vi "PH_Sequencer.Switch PU FR on automatically.vi"(0 "i ref in":refnum<vi>, 5 "error in":errorcluster) -> (14 "i ref out":refnum<vi>, 19 "error out":errorcluster)   [LabVIEW 2014, in "PH_Sequencer.lvlib"]
doc: "This is the action done when PU SM States are changing."
uses:
  PH_Sequencer.lvlib
  PH_PP_Common/PH_PP_Common.PUs.ctl
  PH_BeamlineInformation/PH_BeamlineInformation.lvlib
  PH_PP_Common/PH_PP_Common.lvlib
  PH_PowerUnit_BaseClass/PH_PowerUnit_BaseClass.lvlib
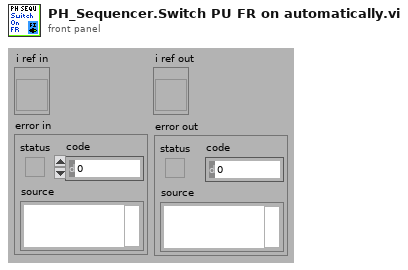
[diagram p1: front panel]
types:
  T1 = typedef "PH_PP_Common.lvlib/PH_PP_Common.PUs.ctl" = enum16{"no Info", "PA-19mm-1", "PA-19mm-2", "PA-45mm-PILC", "PA-45mm-MAIN", "MA-PU-1", "MA-PU-2", "MA-PU-3", "MA-PU-4", "MA-PU-5", "MA-PU-6", "MA-FR", "MA-PILC", "PA-45mm-DP"}
  T2 = typedef "PH_BeamlineInformation.lvlib/PH_BeamlineInformation.i attribute.ctl" = cluster{"BL GUI Elements of Services":cluster{"Service Name":string, "GUI Elements":refnum<vi>[], "Status":i32}[], "Powermeters":T3, "Efficiency":T4, "Heads":T5[]}
  T3 = typedef "PH_BeamlineInformation.lvlib/PH_BeamlineInformation.Powermeter.ctl" = cluster{"ns FE":cluster{"GUI Ref":refnum<vi>, "Value":dbl}, "fs FE":cluster{"GUI Ref":refnum<vi>, "Value":dbl}, "PA":cluster{"GUI Ref":refnum<vi>, "Value":dbl}, "MA":cluster{"GUI Ref":refnum<vi>, "Value":dbl}, "Z6 green":cluster{"GUI Ref":refnum<vi>, "Value":dbl}, "Z6 IR":cluster{"GUI Ref":refnum<vi>, "Value":dbl}, "Z6 COS":cluster{"GUI Ref":refnum<vi>, "Value":dbl}}
  T4 = typedef "PH_BeamlineInformation.lvlib/PH_BeamlineInformation.Efficiency.ctl" = cluster{"PA Gain":cluster{"GUI Ref":refnum<vi>, "Value":dbl}, "MA Gain":cluster{"GUI Ref":refnum<vi>, "Value":dbl}, "Z6 green Conversion":cluster{"GUI Ref":refnum<vi>, "Value":dbl}, "Z6 Comp Losses":cluster{"GUI Ref":refnum<vi>, "Value":dbl}}
  T5 = typedef "PH_BeamlineInformation.lvlib/PH_BeamlineInformation.Head.ctl" = cluster{"PowerUnit":T1, "in use":cluster{"Value":bool, "GUI Ref":refnum<vi>, "linked":bool}, "voltage":cluster{"Value":dbl, "GUI Ref":refnum<vi>, "linked":bool}}
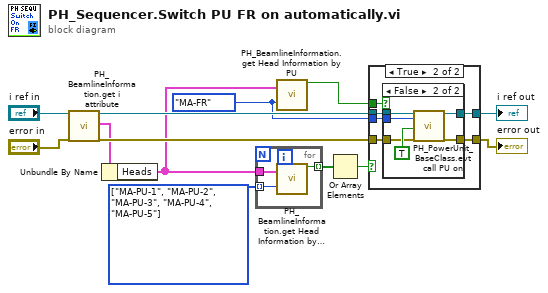
[diagram p0: block diagram]
diagram:
  w1 = PH_PP_Common.PUs."MA-FR" ("Power Unit")
  w6 = T1[] [enum."MA-PU-1", enum."MA-PU-2", enum."MA-PU-3", enum."MA-PU-4", enum."MA-PU-5"] items=["no Info", "PA-19mm-1", "PA-19mm-2", "PA-45mm-PILC", "PA-45mm-MAIN", "MA-PU-1", "MA-PU-2", "MA-PU-3", "MA-PU-4", "MA-PU-5", "MA-PU-6", "MA-FR", "MA-PILC", "PA-45mm-DP"]
  n1 = call "PH_BeamlineInformation.get i attribute.vi"("i ref in"="i ref in", "error in (no error)"="error in") -> ("i ref out"=w8:refnum<vi>, "i attribute"=w7:T2, "error out"=w9:errorcluster)  [unwired: 15 in]
  n2 = Unbundle By Name(w7) -> ("Heads"=w5:T5[])
  n3 = for {
    tunnel: [w14] -> w13 mode=indexing
    tunnel: w5 -> [w16]
    tunnel: w6 -> [w15] mode=indexing
    n4 = call "PH_BeamlineInformation.get Head Information by PU.vi"("Heads"=w16, "Power Unit"=w15) -> ("In Use?"=w14:bool)  [unwired: 12 in, 5 out]
  }
  n5 = call "PH_BeamlineInformation.get Head Information by PU.vi"("Heads"=w5, "Power Unit"=w1) -> ("In Use?"=w4:bool)  [unwired: 12 in, 5 out]
  n6 = Or Array Elements(Boolean array=w13) -> (logical OR=w12:bool)
  n7 = case shown="True" w12 {
    tunnel: w8 -> [w18 w24]
    tunnel: w9 -> [w17 w23]
    tunnel: w4 -> [_ w22]
    tunnel: [w18 w21] -> w11
    tunnel: [w17 w20] -> w10
    tunnel: w1 -> [_ w19]
    frame False {
    }
    frame True {
      n8 = case "Proccase" shown="False" w22 {
        tunnel: [w26 w29] -> w21
        tunnel: w23 -> [w25 w30]
        tunnel: [w25 w28] -> w20
        tunnel: w24 -> [w26 w32]
        tunnel: w19 -> [_ w27]
        frame True {
        }
        frame False {
          n9 = call "PH_PowerUnit_BaseClass.evt call PU on.vi"("i ref in"=w32, "PowerUnit"=w27, "PU on"=TRUE ("PP PU on"), "error in (no error)"=w30) -> ("i ref out"=w29:refnum<vi>, "error out"=w28:errorcluster)  [unwired: 14 in]
        }
      }
    }
  }
  "error out" <- w10
  "i ref out" <- w11
